vi "checkIfTypedefInOldLibrary.vi"(8 "error in (no error)":errorcluster, 10 "specific class reference":refnum<vi>, 11 "Constant in":refnum<class "Constant.lvclass">) -> (0 "error out":errorcluster, 1 "Typedef VI Reference":refnum<vi>, 2 "isMemberOfOldLibrary":bool, 3 "Constant out":refnum<class "Constant.lvclass">)   [LabVIEW 2016, in "Constant.lvclass"]
uses:
  Constant.lvclass
  C:/LSST_TS/SystemSW/ct_tools/GObject/GObject.lvclass
  GObject/GObject.lvclass/GObject.ctl
  Search/Search.lvclass/Search.ctl
  Search/Search.lvclass
  GObject/GObject.lvclass
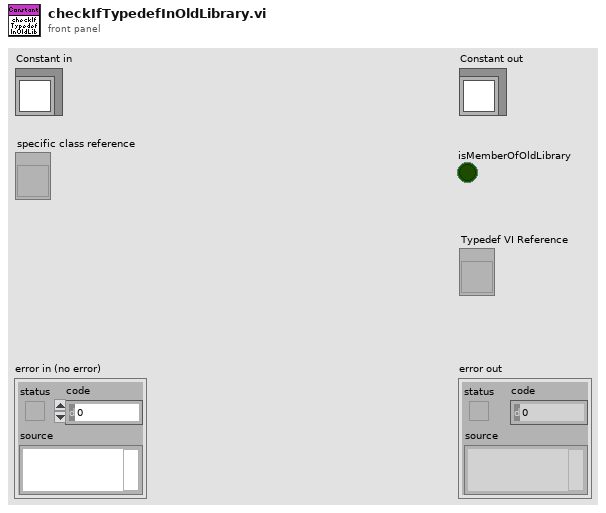
[diagram p1: front panel]
types:
  T1 = cluster{"OldLibrary":string, "NewLibrary":string}
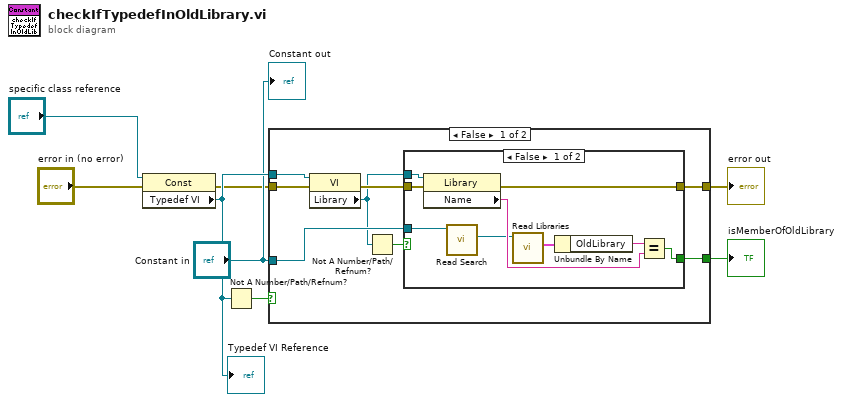
[diagram p0: block diagram]
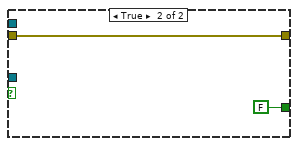
[diagram p2: hidden frame]
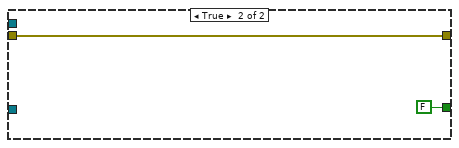
[diagram p3: hidden frame]
diagram:
  n1 = property class="Const"(reference="specific class reference", error in="error in (no error)") -> (error out=w1:errorcluster, "Typedef VI"=w6:refnum<vi>)  [unwired: 1 out]
  "Typedef VI Reference" <- w6
  n2 = Not A Number/Path/Refnum?(number/path/refnum=w6) -> (NaN/Path/Refnum?=w7:bool)
  n3 = case shown="False" w7 {
    tunnel: "Constant in" -> [w16 _]
    tunnel: [w15 FALSE] -> w4
    tunnel: w1 -> [w14 w28]
    tunnel: [w12 w28] -> w3
    tunnel: w6 -> [w9 _]
    frame False {
      n4 = property class="VI"(reference=w9, error in=w14) -> (error out=w13:errorcluster, "Library"=w11:refnum<vi>)  [unwired: 1 out]
      n5 = Not A Number/Path/Refnum?(number/path/refnum=w11) -> (NaN/Path/Refnum?=w10:bool)
      n6 = case shown="False" w10 {
        tunnel: w16 -> [w19 _]
        tunnel: [w23 FALSE] -> w15
        tunnel: w13 -> [w22 w26]
        tunnel: [w21 w26] -> w12
        tunnel: w11 -> [w20 _]
        frame False {
          n7 = property class="Library"(reference=w20, error in=w22) -> (error out=w21:errorcluster, "Name"=w24:string)  [unwired: 1 out]
          n8 = call "Read Search.vi"("DiagramObject in"=w19) -> ("Search.lvclass"=w18:refnum<class "Search.lvclass">)  [unwired: 9 in, 1 out]
          n9 = call "Read Libraries.vi"("ProjectItem in"=w18) -> ("Libraries"=w17:T1)  [unwired: 9 in, 1 out]
          n10 = Unbundle By Name(w17) -> ("OldLibrary"=w25:string)
          n11 = Equal?(x=w25, y=w24) -> (x = y?=w23:bool)
        }
        frame True {
        }
      }
    }
    frame True {
    }
  }
  "error out" <- w3
  "isMemberOfOldLibrary" <- w4
  "Constant out" <- "Constant in"
